vi "SPA_Hex.vi"(0 "System no.":i32=1 min=1 max=4 step=1, 2 "Designator to set":string[](array[string]), 3 "Parameter value":dbl[](array[numeric]) format="%.6f", 4 "No.of digits":i16=4, 5 "error in":errorcluster, 6 "Parameter number (hex)":u32[](array[numeric]) format="%.0x") -> (14 "Controller error":bool, 19 "error out":errorcluster)   [LabVIEW 2026]
doc: "Sets parameters in hex format for commanded designators, waits 100 ms and queries ERR?. See system manual for available parameter numbers and values. No. of digits is the number of digits after the decimal point in the parameter value(s) that will be sent. For axis-related parameters, Designator to set is the axis name; for piezo- or sensor-related parameters, the channel number, otherwise a parameter-related one. Controller error is TRUE if selected system reports an error code which is not 0. \nOld VI - please use SPA.vi instead. \n\nE-710:\nPlease refer to the GCS DLL manual for valid parameter numbers and the stage manual for valid parameter settings. \n\nE-761:\nPlease refer to the GCS DLL manual for valid parameter numbers and the stage manual for valid parameter settings."
panel:
  # "This vi sets parameters in hex format for commanded designators, waits 100 ms and \nqueries ERR?. See GCS DLL manual for available parameter numbers and values.\nOld VI - please use SPA.vi instead."
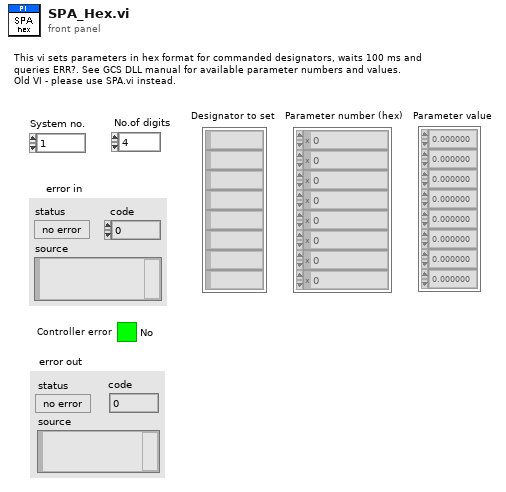
[diagram p1: front panel]
types:
  T1 = enum16{"Disable error check", "Force error check", "Use global settings"}
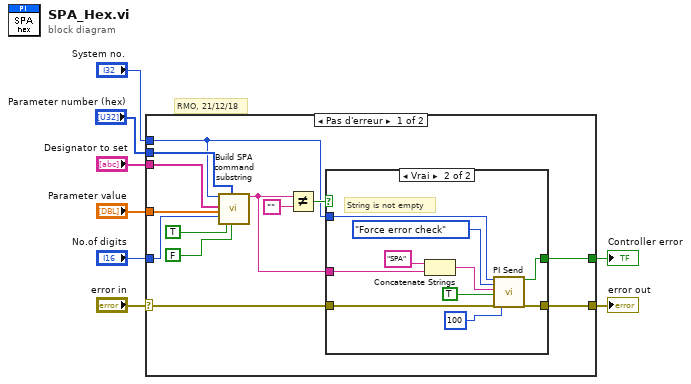
[diagram p0: block diagram]
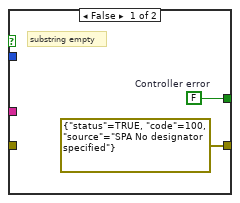
[diagram p2: hidden frame]
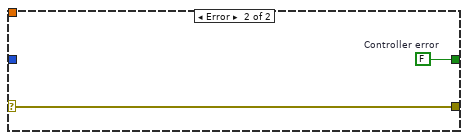
[diagram p3: hidden frame]
diagram:
  # "RMO, 21/12/18"
  n1 = case shown="Pas d'erreur" "error in" {
    selector: "error in" -> [w10 w35]
    tunnel: [w21 w35] -> w8
    tunnel: "Parameter value" -> [w18 _]
    tunnel: "No.of digits" -> [w17 _]
    tunnel: "System no." -> [w13 _]
    tunnel: "Designator to set" -> [w16 _]
    tunnel: "Parameter number (hex)" -> [w15 _]
    tunnel: [w9 w34] -> w1
    frame No Error {
      n2 = call "Build SPA command substring.vi"("System no."=w13, "Axes to set"=w16, "Parameter values"=w18, "No. of digits"=w17, "Parameter no. format \n(Decimal: FALSE)"=TRUE ("Parameter no. format \n(Decimal: FALSE)"), "Parameter number (hex)"=w15, "Parameter format \n(Num.: FALSE)"=FALSE ("Parameter format \n(Num.: FALSE)")) -> ("SPA command substring"=w19:string)  [unwired: 3 in, 9 out]
      n3 = Not Equal?(x=w19, y="") -> (x != y?=w14:bool)
      n4 = case shown="Vrai" w14 {
        tunnel: w19 -> [_ w32]
        tunnel: [errorcluster {"status"=TRUE, "code"=100, "source"="SPA No designator specified"} ("error out") w26] -> w21
        tunnel: w10 -> [_ w29]
        tunnel: w13 -> [_ w28]
        tunnel: [w22 w24] -> w9
        frame False {
          w22 = FALSE  # Controller error
          # "substring empty"
        }
        frame True {
          # "String is not empty"
          n5 = Concatenate Strings("SPA", w32) -> (w30:string)
          n6 = call "PI Send.vi"("System no."=w28, "Error check settings"=T1."Force error check", "String to send"=w30, "Attach termination char.?"=TRUE ("Attach Linefeed?"), "error in"=w29, "Delay before error check (ms)"=u32 100 ("milliseconds to wait")) -> ("Controller error"=w24:bool, "error out"=w26:errorcluster)  [unwired: 12 out]
        }
      }
    }
    frame Error {
      w34 = FALSE  # Controller error
    }
  }
  "error out" <- w8
  "Controller error" <- w1
